vi "subtract.vi"(8 "error in (no error)":errorcluster, 10 "subtrahend":refnum<class "ImageCollection.lvclass">, 11 "ImageCollection in":refnum<class "ImageCollection.lvclass">) -> (0 "error out":errorcluster, 3 "ImageCollection out":refnum<class "ImageCollection.lvclass">)   [LabVIEW 2010, in "ImageCollection.lvclass"]
uses:
  ImageCollection.lvclass
  Image/Image/Image.lvclass
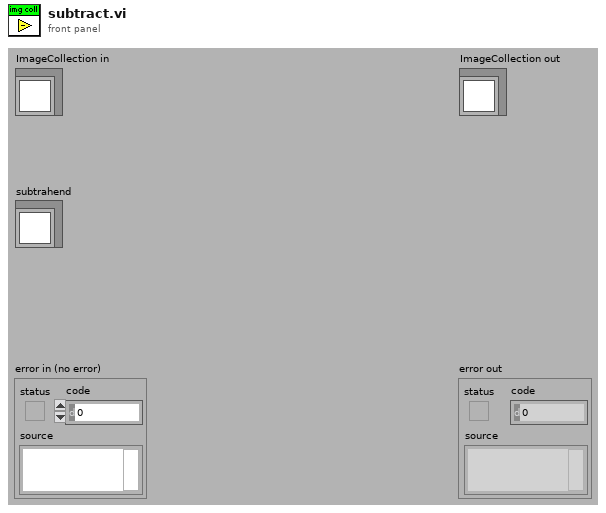
[diagram p1: front panel]
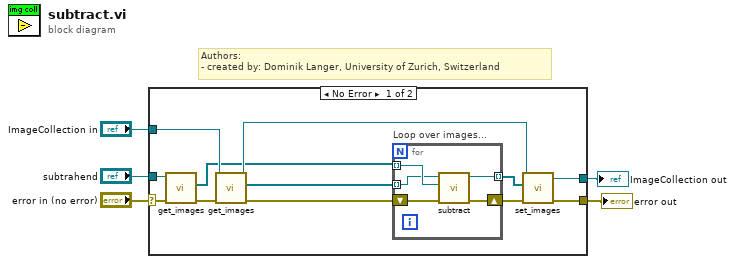
[diagram p0: block diagram]
diagram:
  # "Authors: \n- created by: Dominik Langer, University of Zurich, Switzerland"
  n1 = case shown="No Error" "error in (no error)" {
    selector: "error in (no error)" -> [w16 w24]
    tunnel: [w11 w24] -> w4
    tunnel: [w9 w23] -> w2
    tunnel: "ImageCollection in" -> [w17 w23]
    tunnel: "subtrahend" -> [w14 _]
    frame No Error {
      n2 = call-dynamic "get_images.vi"("error in (no error)"=w16, "ImageCollection.lvclass in"=w14) -> ("error out"=w15:errorcluster, "images"=w7:refnum<class "Image.lvclass">[])  [unwired: 8 out]
      n3 = call-dynamic "get_images.vi"("error in (no error)"=w15, "ImageCollection.lvclass in"=w17) -> ("error out"=w8:errorcluster, "images"=w6:refnum<class "Image.lvclass">[], "ImageCollection.lvclass out"=w10:refnum<class "ImageCollection.lvclass">)  [unwired: 7 out]
      n4 = for "Loop over images..." {
        tunnel: w6 -> [w20] mode=indexing
        tunnel: w7 -> [w21] mode=indexing
        shift-right: [w18] -> w13
        shift-left: w8 -> [w22]
        tunnel: [w19] -> w12 mode=indexing
        n5 = call-dynamic "subtract.vi"("error in (no error)"=w22, "subtrahend"=w21, "Image in"=w20) -> ("error out"=w18:errorcluster, "Image out"=w19:refnum<class "Image.lvclass">)  [unwired: 7 out]
      }
      n6 = call-dynamic "set_images.vi"("error in (no error)"=w13, "images"=w12, "ImageCollection.lvclass in"=w10) -> ("error out"=w11:errorcluster, "ImageCollection.lvclass out"=w9:refnum<class "ImageCollection.lvclass">)  [unwired: 7 out]
    }
    frame Error {
    }
  }
  "error out" <- w4
  "ImageCollection out" <- w2
